vi "GetImage.vi"(8 "error in (no error)":errorcluster, 9 "Header Info In":string, 11 "connection ID in":refnum<k5>) -> (0 "error out":errorcluster, 1 "JPEG File?":bool, 2 "Image/Movie Out":T1 {"Dialogs" format="%.0b"}, 3 "connection ID":refnum<k5>, 4 "picture out TEST":picture, 6 "dimensions":cluster{"Width":i32, "Height":i32})   [LabVIEW 2014]
uses:
  ImageProcessing/QT_Image.ctl
panel:
  in  "Image Setting":T1 {"Dialogs" format="%.0b"}
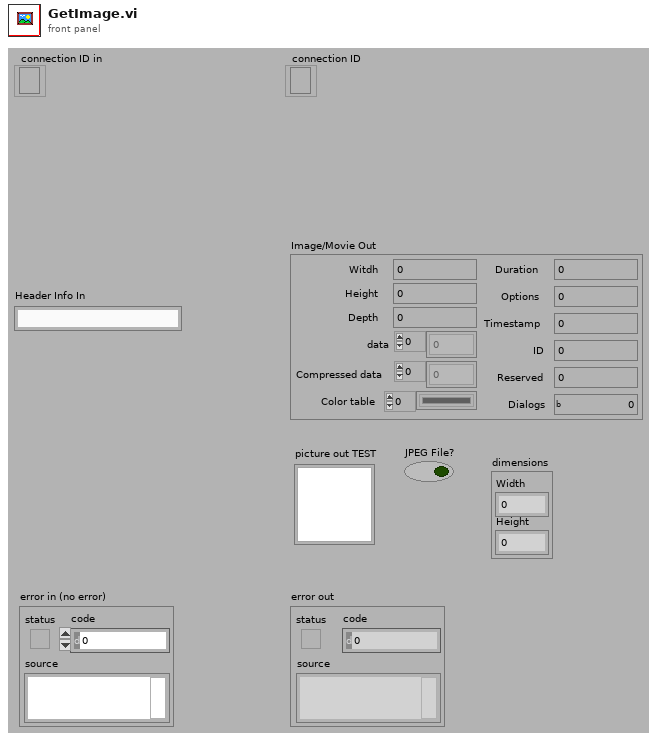
[diagram p1: front panel]
types:
  T1 = typedef "QT_Image.ctl" = cluster{"Witdh":i32, "Height":i32, "Depth":i32, "data":u8[], "Compressed data":u8[], "Color table":u32[], "Duration":i32, "Options":i32, "Timestamp":i32, "ID":i32, "Reserved":i32, "Dialogs":u32}
  T2 = enum16{"big-endian, network order", "native, host order", "little-endian"}
  T3 = typedef "imagedata.ctl" = cluster{"image type":i32, "image depth":i32, "image":u8[], "mask":u8[], "colors":u32[], "Rectangle":cluster{"left":i16, "top":i16, "right":i16, "bottom":i16}}
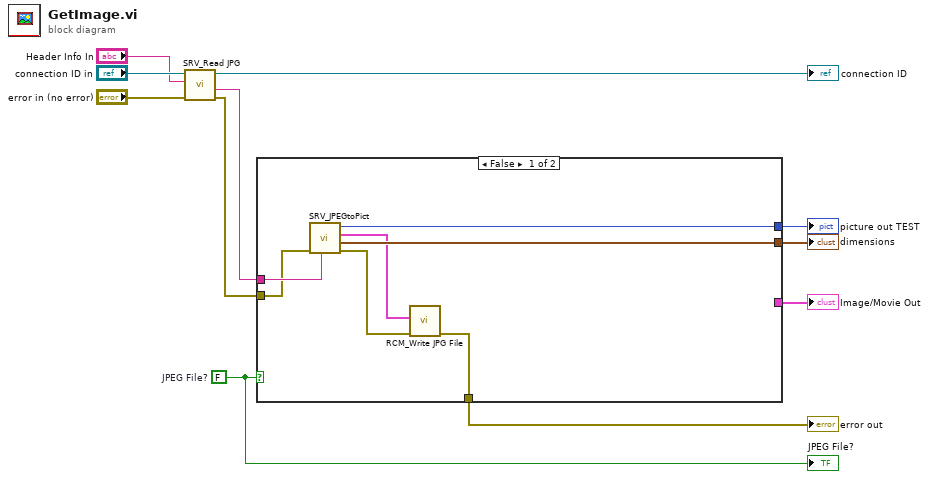
[diagram p0: block diagram]
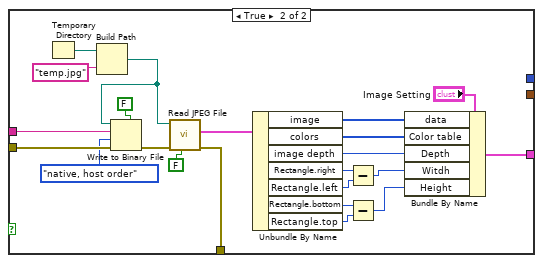
[diagram p2: hidden frame]
diagram:
  w3 = FALSE  # JPEG File?
  n1 = call "SRV_Read JPG.vi"("error in"="error in (no error)", "Header Info In"="Header Info In", "connection ID in"="connection ID in") -> ("error out"=w9:errorcluster, "data out"=w4:string, "connection ID"=→"connection ID":refnum<k5>)  [unwired: 6 in]
  n2 = case shown="False" w3 {
    tunnel: [_ w40] -> w11
    tunnel: w9 -> [w17 w39]
    tunnel: [w12 w38] -> w8
    tunnel: w4 -> [w18 w19]
    tunnel: [w16 _] -> w2
    tunnel: [w15 _] -> w1
    frame False {
      n3 = call "SRV_JPEGtoPict.vi"("jpeg string"=w18, "error in (no error)"=w17) -> ("error out"=w13:errorcluster, "dimensions"=w15:cluster{"Width":i32, "Height":i32}, "image data"=w14:T3, "picture out"=w16:picture)  [unwired: 6 in]
      n4 = call "RCM_Write JPG File.vi"("error in (no error)"=w13, "image data"=w14) -> ("error out"=w12:errorcluster)  [unwired: 9 in]
    }
    frame True {
      n5 = Temporary Directory() -> (w20:path)
      n6 = Build Path(base path=w20, name or relative path="temp.jpg") -> (appended path=w35:path)
      n7 = Write to Binary File(file (use dialog)=w35, data=w19, error in=w39, 5:FALSE ("prepend array or string size? (T)"), 9:T2."native, host order" ("byte order (0:big-endian, network order)")) -> (error out=w36:errorcluster)  [unwired: 1 in, 2 out]
      n8 = call <vilib>:"Read JPEG File.vi"("use 8 bit color table"=FALSE, "error in (no error)"=w36, "path to JPEG file"=w35) -> ("error out"=w38:errorcluster, "image data"=w34:T3)  [unwired: 6 in, 1 out]
      n9 = Unbundle By Name(w34) -> ("image"=w33:u8[], "colors"=w32:u32[], "image depth"=w31:i32, "Rectangle.right"=w30:i16, "Rectangle.left"=w29:i16, "Rectangle.bottom"=w26:i16, "Rectangle.top"=w25:i16)
      n10 = Subtract(x=w30, y=w29) -> (x-y=w28:i16)
      n11 = Subtract(x=w26, y=w25) -> (x-y=w27:i16)
      n12 = Bundle By Name(cluster="Image Setting", "data"=w33, "Color table"=w32, "Depth"=w31, "Witdh"=w28, "Height"=w27) -> (w40:T1)
    }
  }
  "Image/Movie Out" <- w11
  "error out" <- w8
  "picture out TEST" <- w2
  "dimensions" <- w1
  "JPEG File?" <- w3
